vi "Init Msg Output.vi"() -> (3 "Stop Msg Output out":refnum<class "Stop Msg Output.lvclass">)   [LabVIEW 2025, in "jettl.lvlib" / "Stop jettl Msg.lvlib" / "Stop Msg Output.lvlib" / "Stop Msg Output.lvclass"]
uses:
  Stop Msg Output.lvclass
  Stop Msg Output.lvclass/Stop Msg Output.ctl
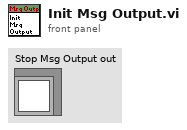
[diagram p1: front panel]
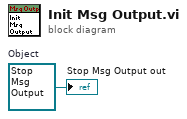
[diagram p0: block diagram]
diagram:
  w1 = refnum<class "Stop Msg Output.lvclass"> refnum  # Object
  "Stop Msg Output out" <- w1
